vi "SubVI_SolenoidFire_Teleop.vi"(11 "Solenoid":string="My Solenoid RefNum") -> ()   [LabVIEW 2017]
uses:
  <vilib>/Rock Robotics/WPI/Solenoid/WPI_SolenoidValue.ctl
  <vilib>/Rock Robotics/WPI/Solenoid/WPI_SolenoidSetEnum.vi
panel:
  in  "error in (no error)":errorcluster
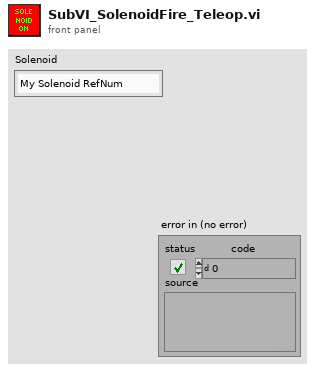
[diagram p1: front panel]
types:
  T1 = typedef "WPI_SolenoidValue.ctl" = enum16{"Off", "On", "Forward", "Reverse"}
  T2 = typedef "WPI_SolenoidDevRef.ctl" = cluster{"DevStatus":errorcluster, "Pneumatics Control Module":u8, "Forward Solenoid Channel":T3, "Reverse Solenoid Channel":T3}
  T3 = typedef "WPI_SolenoidChannel.ctl" = enum8{"Solenoid 0", "Solenoid 1", "Solenoid 2", "Solenoid 3", "Solenoid 4", "Solenoid 5", "Solenoid 6", "Solenoid 7", "Invalid"}
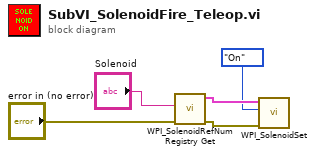
[diagram p0: block diagram]
diagram:
  n1 = call <vilib>:"WPI_SolenoidRefNum Registry Get.vi"("error in (no error)"="error in (no error)", "refnum name"="Solenoid") -> ("error out"=w5:errorcluster, "SolenoidDevRef"=w4:T2)  [unwired: 8 in]
  n2 = call-poly <vilib>:"WPI_SolenoidSet.vi"("error in (no error)"=w5, "Value"=WPI_SolenoidValue."On", "SolenoidDevRef"=w4) -> ()  [unwired: 7 in, 2 out]
